vi "Root Location Global.vi"() -> ()   [LabVIEW 2011]
panel:
  in  "root":path
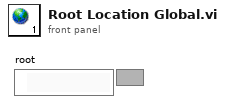
[diagram p1: front panel]
diagram:
